vi "MTMount_getSample_MainPowerSupplyCabinet.vi"(8 "error in (no error)":errorcluster, 11 "Main_Power_Supply_Cabinet_Ctl":T1) -> (0 "error out":errorcluster, 2 "function return":i32, 3 "Main_Power_Supply_Cabinet_Ctl out":T1)   [LabVIEW 2018, in "SALLV_MTMount.lvlib"]
doc: "int MTMount_shm_getSample_Main_Power_Supply_CabinetLV(MTMount_Main_Power_Supply_CabinetLV *Main_Power_Supply_Cabinet_Ctl );"
uses:
  SALLV_MTMount.lvlib
  DataTypes/Main_Power_Supply_Cabinet.ctl
  SALLV_MTMount.so
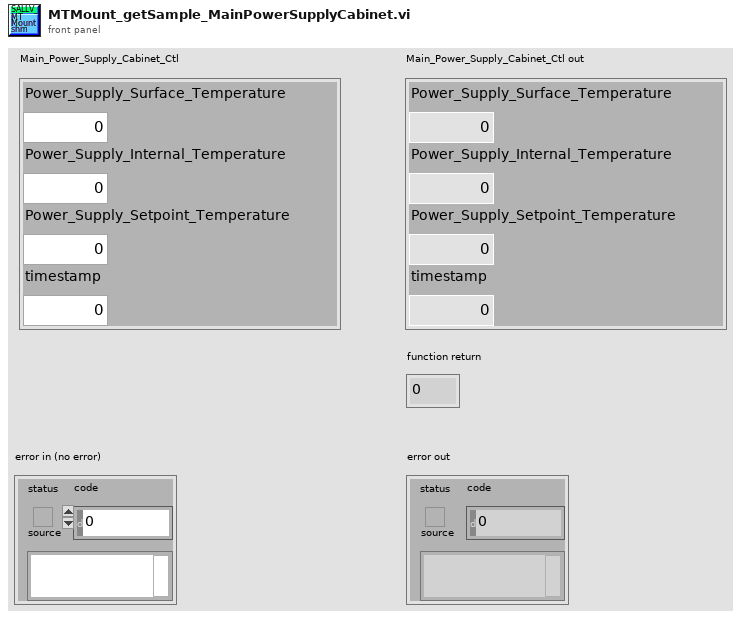
[diagram p1: front panel]
types:
  T1 = typedef "SALLV_MTMount.lvlib/Main_Power_Supply_Cabinet.ctl" = cluster{"Power_Supply_Surface_Temperature":dbl, "Power_Supply_Internal_Temperature":dbl, "Power_Supply_Setpoint_Temperature":dbl, "timestamp":dbl}
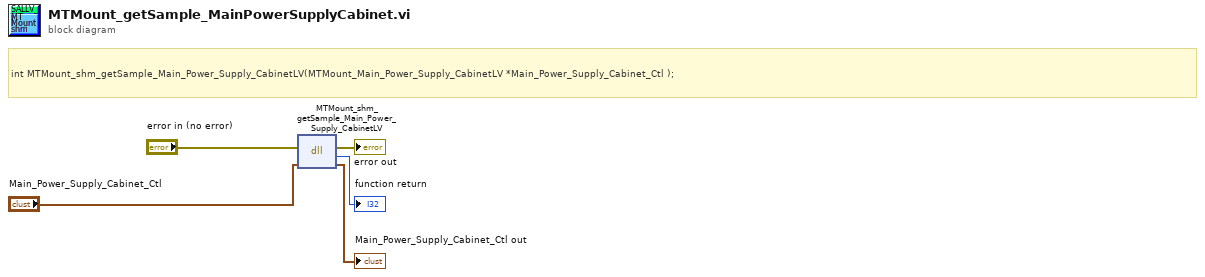
[diagram p0: block diagram]
diagram:
  # "int MTMount_shm_getSample_Main_Power_Supply_CabinetLV(MTMount_Main_Power_Supply_CabinetLV *Main_Power_Supply_Cabinet_Ctl );"
  n1 = dll-call lib="home/ttsai/Document/salApiMTMount/SALLV_MTMount/SALLV_MTMount.*" fn="MTMount_shm_getSample_Main_Power_Supply_CabinetLV"(error in="error in (no error)", "Main_Power_Supply_Cabinet_Ctl"="Main_Power_Supply_Cabinet_Ctl") -> (error out=→"error out":errorcluster, →"function return":i32, "Main_Power_Supply_Cabinet_Ctl"=→"Main_Power_Supply_Cabinet_Ctl out":T1)  [unwired: 2 in, 1 out]
